vi "BTW_Visual_Database_Ops.vi"(8 "Error in (no error)":errorcluster, 10 "Old server? (n)":bool, 11 "SQL Query":string) -> (0 "Error out":errorcluster, 2 "Rec Count":i32, 3 "RecordSet":string[][](array[string]))   [LabVIEW 2013]
uses:
  Test Globals/Global 1.vi
panel:
  out "VisualSqlConnStr":string="DRIVER=SQL Server;SERVER=BTWSQLSERVER1;DATABASE=VMFG;UID=BTW_USER;PWD=mbfFMz6LJpWk3ABm"
  in  "Record data":string[](array[string])
  out "Column Names":string[](array[string])
  in  "Operation":T1(ring)=enum."Select"
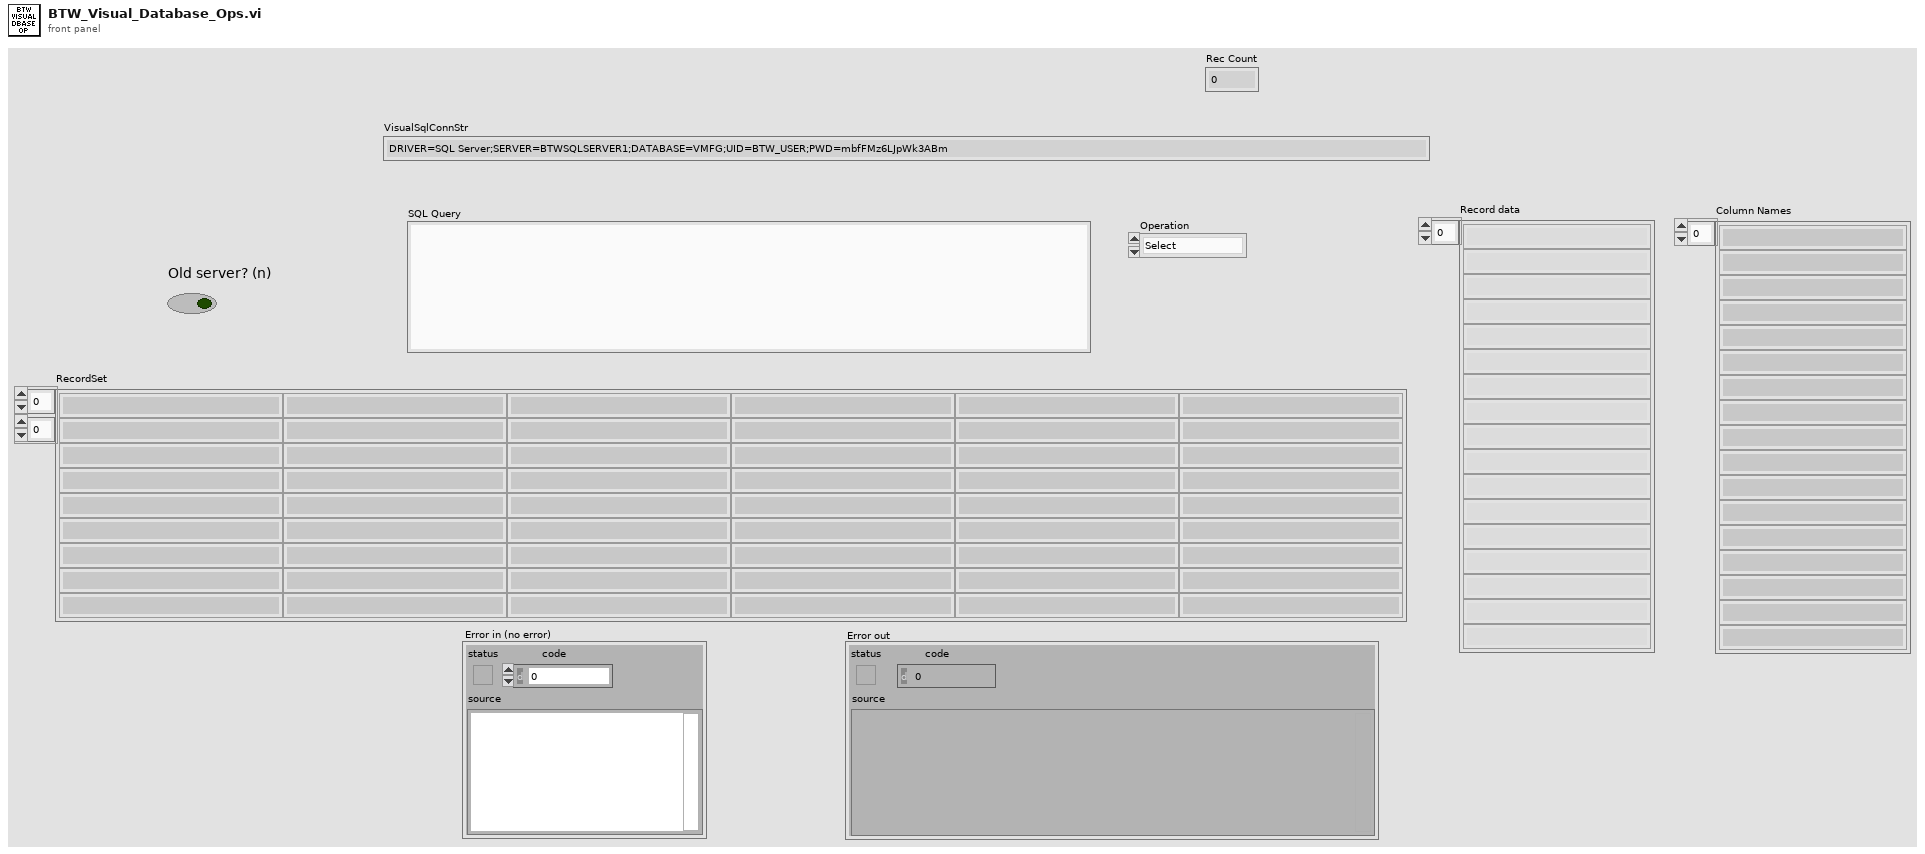
[diagram p1: front panel]
types:
  T1 = enum16{"Query", "Insert", "Select", "Dump Recs", "Get Rec Count", "Get Col Names"}
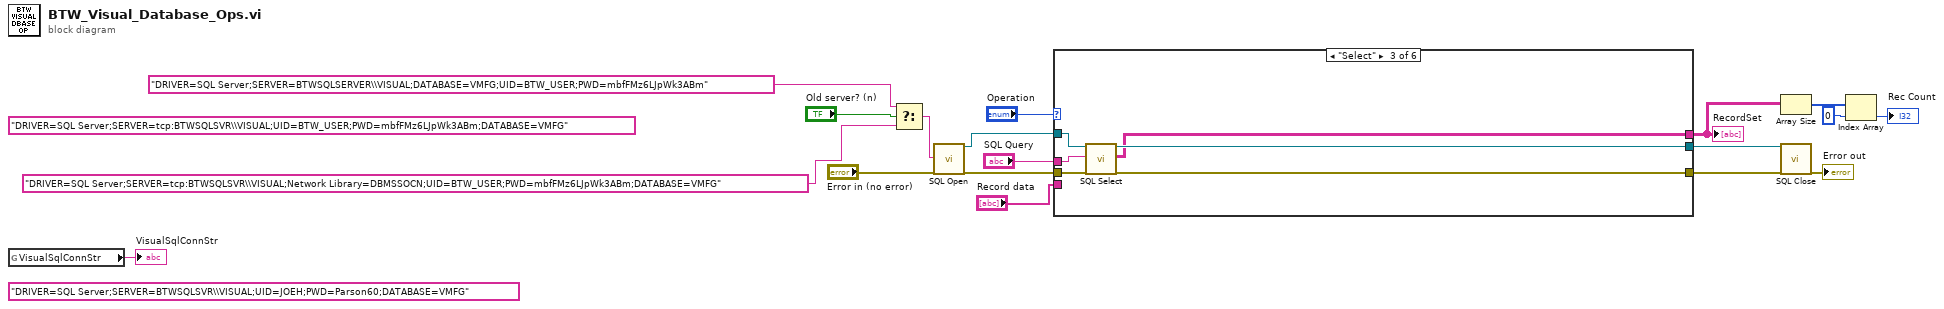
[diagram p0: block diagram]
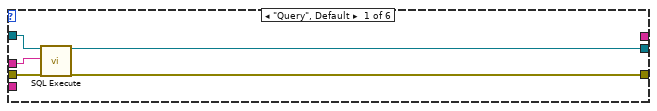
[diagram p2: hidden frame]
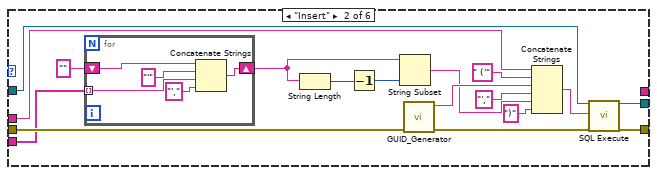
[diagram p3: hidden frame]
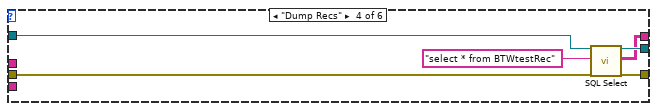
[diagram p4: hidden frame]
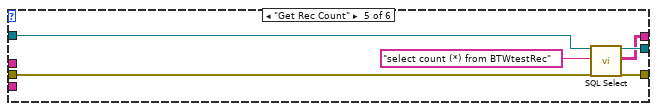
[diagram p5: hidden frame]
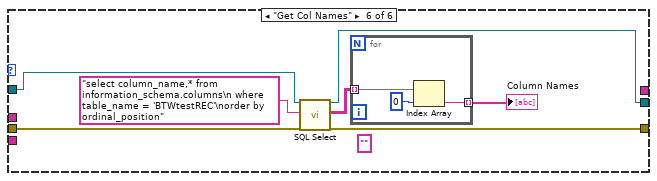
[diagram p6: hidden frame]
diagram:
  (unwired) "DRIVER=SQL Server;SERVER=BTWSQLSVR\\VISUAL;UID=JOEH;PWD=Parson60;DATABASE=VMFG"
  (unwired) "DRIVER=SQL Server;SERVER=tcp:BTWSQLSVR\\VISUAL;UID=BTW_USER;PWD=mbfFMz6LJpWk3ABm;DATABASE=VMFG"
  n1 = global read "Global 1.vi" "VisualSqlConnStr"() -> (→"VisualSqlConnStr":string)
  n2 = Select(t="DRIVER=SQL Server;SERVER=BTWSQLSERVER\\VISUAL;DATABASE=VMFG;UID=BTW_USER;PWD=mbfFMz6LJpWk3ABm", s="Old server? (n)", f="DRIVER=SQL Server;SERVER=tcp:BTWSQLSVR\\VISUAL;Network Library=DBMSSOCN;UID=BTW_USER;PWD=mbfFMz6LJpWk3ABm;DATABASE=VMFG") -> (s? t:f=w2:string)
  n3 = call "SQL Open.vi"("ConnectionString In"=w2, "Error in (no error)"="Error in (no error)") -> ("Connection Out"=w15:refnum<k7>, "Error out"=w14:errorcluster)  [unwired: 16 in]
  n4 = case shown="\"Select\"" "Operation" {
    tunnel: [w20 w40 w47 w54 w59 w65] -> w17
    tunnel: [w19 w39 w48 w55 w60 w64] -> w16
    tunnel: w15 -> [w22 w38 w49 w57 w63 w69]
    tunnel: w14 -> [w21 w37 w51 w56 w62 w68]
    tunnel: "SQL Query" -> [w23 w31 w50 _ _ _]
    tunnel: [_ _ w46 w52 w58 _] -> w8
    tunnel: "Record data" -> [_ w36 _ _ _ _]
    frame "Query", Default {
      n5 = call "SQL Execute.vi"("Connection In"=w22, "SQL Query"=w23, "Error in (no error)"=w21) -> ("Connection Out"=w19:refnum<k7>, "Error out"=w20:errorcluster)  [unwired: 15 in]
    }
    frame "Insert" {
      n6 = for {
        tunnel: w36 -> [w45] mode=indexing
        shift-right: [w43] -> w25
        shift-left: "" -> [w42]
        n7 = Concatenate Strings(w42, "'" ("string"), w45, "'," ("string")) -> (w43:string)
      }
      n8 = String Length(string=w25) -> (length=w27:i32)
      n9 = Decrement(x=w27) -> (x-1=w26:i32)
      n10 = String Subset(string=w25, length (rest)=w26) -> (substring=w24:string)  [unwired: 1 in]
      n11 = call "GUID_Generator.vi"("error in (no error)"=w37) -> ("error out"=w29:errorcluster, "GUID String"=w35:string)  [unwired: 9 in]
      n12 = Concatenate Strings(w31, " ('" ("string"), w35, "'," ("string"), w24, ")") -> (w30:string)
      n13 = call "SQL Execute.vi"("Connection In"=w38, "SQL Query"=w30, "Error in (no error)"=w29) -> ("Connection Out"=w39:refnum<k7>, "Error out"=w40:errorcluster)  [unwired: 15 in]
    }
    frame "Select" {
      n14 = call "SQL Select.vi"("Connection In"=w49, "SQL Query"=w50, "Error in (no error)"=w51) -> ("Connection Out"=w48:refnum<k7>, "Data"=w46:string[][], "Error out"=w47:errorcluster)  [unwired: 14 in]
    }
    frame "Dump Recs" {
      n15 = call "SQL Select.vi"("Connection In"=w57, "SQL Query"="select * from BTWtestRec", "Error in (no error)"=w56) -> ("Connection Out"=w55:refnum<k7>, "Data"=w52:string[][], "Error out"=w54:errorcluster)  [unwired: 14 in]
    }
    frame "Get Rec Count" {
      n16 = call "SQL Select.vi"("Connection In"=w63, "SQL Query"="select count (*) from BTWtestRec", "Error in (no error)"=w62) -> ("Connection Out"=w60:refnum<k7>, "Data"=w58:string[][], "Error out"=w59:errorcluster)  [unwired: 14 in]
    }
    frame "Get Col Names" {
      (unwired) "" ("SQL Query")
      n17 = call "SQL Select.vi"("Connection In"=w69, "SQL Query"="select column_name,* from information_schema.columns\n where table_name = 'BTWtestREC'\norder by ordinal_position", "Error in (no error)"=w68) -> ("Connection Out"=w64:refnum<k7>, "Data"=w67:string[][], "Error out"=w65:errorcluster)  [unwired: 14 in]
      n18 = for {
        tunnel: w67 -> [w73] mode=indexing
        tunnel: [w72] -> w66 mode=indexing
        n19 = Index Array(array=w73, index=0 ("index (col)")) -> (element=w72:string)
      }
      "Column Names" <- w66
    }
  }
  "RecordSet" <- w8
  n20 = Array Size(array=w8) -> (size(s)=w10:i32[])
  n21 = call "SQL Close.vi"("Connection In"=w16, "Error in (no error)"=w17) -> ("Error out"=→"Error out":errorcluster)  [unwired: 17 in]
  n22 = Index Array(array=w10, index=0) -> (element=→"Rec Count":i32)
